vi "SignalGenerator.vi"(7 "error in (no error)":errorcluster, 8 "Stop":bool, 9 "Amplitude":dbl, 10 "Frequency":dbl) -> (2 "error out":errorcluster)   [LabVIEW 2015]
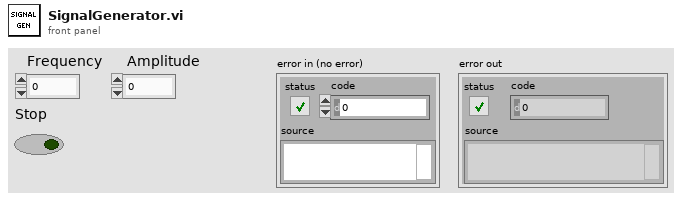
[diagram p1: front panel]
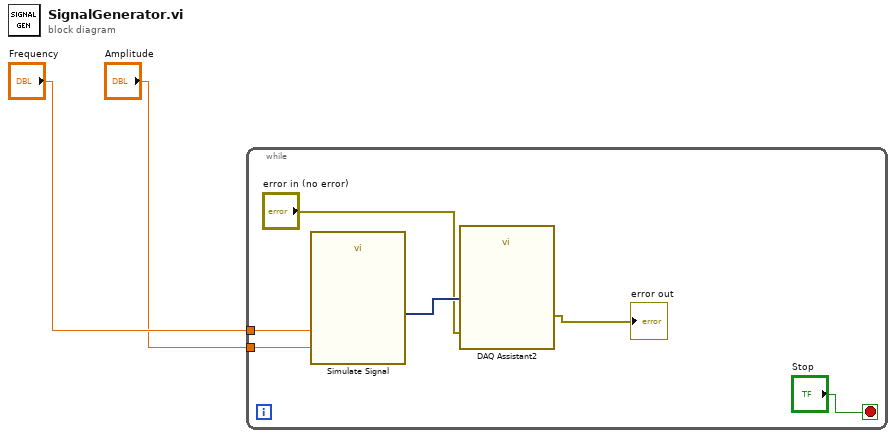
[diagram p0: block diagram]
diagram:
  n1 = while {
    tunnel: "Frequency" -> [w6]
    tunnel: "Amplitude" -> [w5]
    stop <- "Stop" stop-if-true
    n2 = call "Simulate Signal"("Frequency"=w6, "Amplitude"=w5) -> ("Sine"=w7:dynamicdata)  [unwired: 12 in, 1 out]
    n3 = call "DAQ Assistant2"("data"=w7, "error in"="error in (no error)") -> ("error out"=→"error out":errorcluster)  [unwired: 15 in, 2 out]
  }
